vi "dfd_FXP compare.vi"(8 "High 64_2":i64, 9 "Low 64_2":u64, 10 "High 64_1":i64, 11 "Low 64_1":u64) -> (0 "Smaller high64":i64, 1 "Smaller low64":u64, 2 "Bigger high64":i64, 3 "Bigger low64":u64)   [LabVIEW 2017, in "NI_DigFilter_FXP.lvlib"]
uses:
  <vilib>/addons/Digital Filter Design/NI_DigFilter_FXP.lvlib
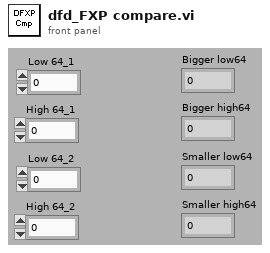
[diagram p1: front panel]
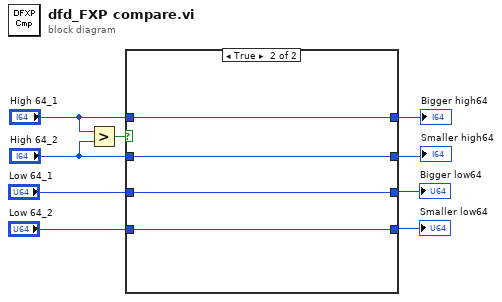
[diagram p0: block diagram]
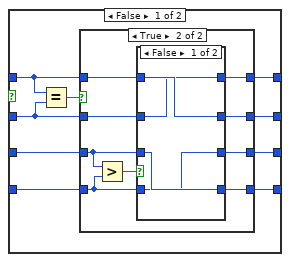
[diagram p2: hidden frame]
diagram:
  n1 = Greater?(x="High 64_1", y="High 64_2") -> (0:w9:bool)
  n2 = case shown="True" w9 {
    tunnel: "High 64_1" -> [w15 w43]
    tunnel: "High 64_2" -> [w14 w42]
    tunnel: "Low 64_1" -> [w17 w41]
    tunnel: "Low 64_2" -> [w16 w40]
    tunnel: [w13 w43] -> w4
    tunnel: [w12 w42] -> w3
    tunnel: [w11 w41] -> w2
    tunnel: [w10 w40] -> w1
    frame False {
      n3 = Equal?(x=w15, y=w14) -> (x = y?=w18:bool)
      n4 = case shown="True" w18 {
        tunnel: w17 -> [w20 w26]
        tunnel: w16 -> [w19 w24]
        tunnel: w15 -> [w22 w30]
        tunnel: w14 -> [w21 w28]
        tunnel: [w21 w29] -> w13
        tunnel: [w22 w27] -> w12
        tunnel: [w19 w25] -> w11
        tunnel: [w20 w23] -> w10
        frame False {
        }
        frame True {
          n5 = Greater?(x=w26, y=w24) -> (0:w31:bool)
          n6 = case shown="False" w31 {
            tunnel: [w34 w39] -> w29
            tunnel: w30 -> [w35 w39]
            tunnel: [w35 w38] -> w27
            tunnel: w28 -> [w34 w38]
            tunnel: [w32 w37] -> w25
            tunnel: w26 -> [w33 w37]
            tunnel: [w33 w36] -> w23
            tunnel: w24 -> [w32 w36]
            frame False {
            }
            frame True {
            }
          }
        }
      }
    }
    frame True {
    }
  }
  "Bigger high64" <- w4
  "Bigger low64" <- w2
  "Smaller high64" <- w3
  "Smaller low64" <- w1
